vi "EventStructure.vi"() -> ()   [LabVIEW 2018]
panel:
  out "Timeout":bool
  in  "?":bool
  in  "?":bool
  # "True"
  # "False"
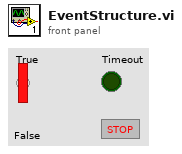
[diagram p1: front panel]
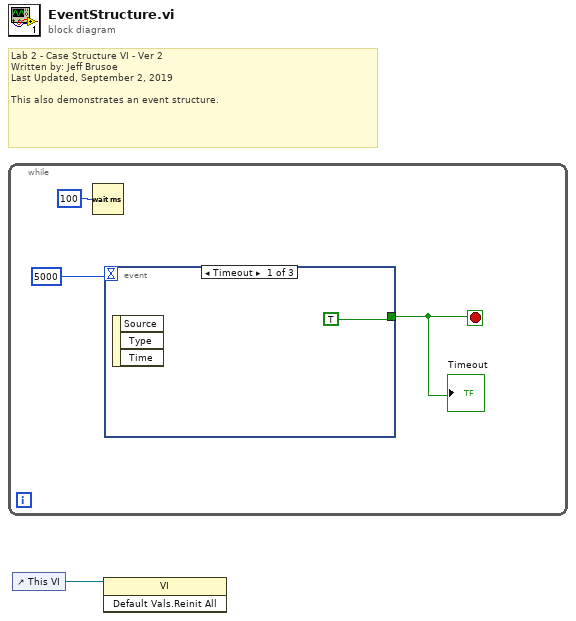
[diagram p0: block diagram]
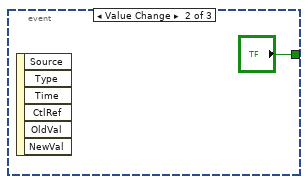
[diagram p2: hidden frame]
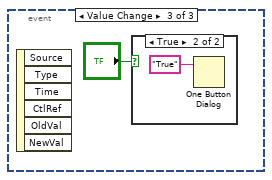
[diagram p3: hidden frame]
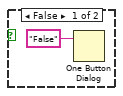
[diagram p4: hidden frame]
diagram:
  # "Lab 2 - Case Structure VI - Ver 2\nWritten by: Jeff Brusoe\nLast Updated, September 2, 2019\n\nThis also demonstrates an event structure."
  n1 = while {
    stop <- w2 stop-if-true
    n2 = Wait (ms)(milliseconds to wait=100) -> ()  [unwired: 1 out]
    n3 = event shown="[0] Timeout" {
      selector: _ -> [_ _ _]
      dyn-events: _ -> [_ _ _]
      timeout: 5000 -> [_ _ _]
      tunnel: [TRUE "?" _] -> w2
      event Timeout {
        n4 = event-data() -> ()  [unwired: 1 in, 3 out]
      }
      event Value Change {
        n5 = event-data() -> ()  [unwired: 1 in, 6 out]
      }
      event Value Change {
        n6 = event-data() -> ()  [unwired: 1 in, 6 out]
        n7 = case shown="True" "?" {
          frame False {
            n8 = One Button Dialog(message="False") -> ()  [unwired: 1 in, 1 out]
          }
          frame True {
            n9 = One Button Dialog(message="True") -> ()  [unwired: 1 in, 1 out]
          }
        }
      }
    }
    "Timeout" <- w2
  }
  n10 = control-ref of="This VI"() -> (w1:refnum<vi>)
  n11 = invoke class="VI" method="Default Vals.Reinit All"(reference=w1) -> ()  [unwired: 2 in, 3 out]
